vi "Remove.vi"(4 "case matching (sensitive)":T1=enum."system", 6 "key":string, 7 "array in":T2) -> (1 "valid key":bool, 2 "value":string, 3 "array out":T2)   [LabVIEW 2015, in "TLB` Template.lvlib" / "Tools_KeyedArray.lvlib"]
doc: "Removes the element identified by <B>key</B> from <B>array in</B>.TLB Prime - Application Template 1.3.0.24\nNorm Kirchner, NI Systems Engineering - NI\nCopyright (c) 2014, NI"
uses:
  Tools_KeyedArray.lvlib
  KeyedArray.ctl
  <vilib>/FTP/util/Case Matching.ctl
  Get Case Matching.vi
  <vilib>/FTP/NI_FTP.lvlib
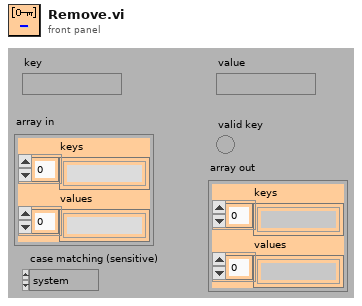
[diagram p1: front panel]
types:
  T1 = typedef "NI_FTP.lvlib/Case Matching.ctl" = enum16{"a != A", "a == A", "system"}
  T2 = typedef "TLB` Template.lvlib/Tools_KeyedArray.lvlib/KeyedArray.ctl" = cluster{"keys":string[], "values":string[]}
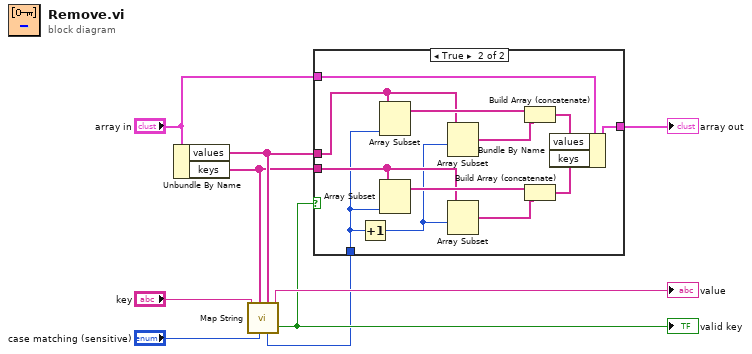
[diagram p0: block diagram]
diagram:
  n1 = Unbundle By Name("array in") -> ("values"=w4:string[], "keys"=w2:string[])
  n2 = call "Map String.vi"("case matching (sensitive)"="case matching (sensitive)", "key"="key", "keys"=w2, "values"=w4) -> ("index"=w3:i32, "valid key"=w7:bool, "value"=→"value":string)  [unwired: 1 in]
  "valid key" <- w7
  n3 = case shown="True" w7 {
    tunnel: "array in" -> [w10 w13]
    tunnel: [w10 w14] -> w5
    tunnel: w4 -> [_ w20]
    tunnel: w3 -> [_ w12]
    tunnel: w2 -> [_ w17]
    frame False {
    }
    frame True {
      n4 = Increment(x=w12) -> (x+1=w11:i32)
      n5 = Array Subset(array=w20, length=w12) -> (w22:string[])  [unwired: 1 in]
      n6 = Array Subset(array=w17, length=w12) -> (w18:string[])  [unwired: 1 in]
      n7 = Array Subset(array=w20, index=w11) -> (w21:string[])  [unwired: 1 in]
      n8 = Array Subset(array=w17, index=w11) -> (w19:string[])  [unwired: 1 in]
      n9 = Build Array (concatenate)(w22, w21) -> (w15:string[])
      n10 = Build Array (concatenate)(w18, w19) -> (w16:string[])
      n11 = Bundle By Name(cluster=w13, "values"=w15, "keys"=w16) -> (w14:T2)
    }
  }
  "array out" <- w5
